vi "Set Batch Text.vi"(0 "VISA resource name":refnum<visa-resource-name>, 5 "Field Number (1)":i32=1 min=1 max=24, 7 "Field Title (\"\")":string, 9 "Field String (\"\")":string, 11 "error in (no error)":errorcluster) -> (4 "VISA resource name out":refnum<visa-resource-name>, 15 "error out":errorcluster)   [LabVIEW 2020, in "Yokogawa GX Series.lvlib"]
doc: "Sets the batch text.\n\nCommand: OBatText"
uses:
  <instrlib>/Yokogawa GX Series/Yokogawa GX Series.lvlib
panel:
  in  "Batch Group Number  (0: OFF)":i32(ring) items=["OFF", "1", "2", "3", "4", "5", "6", "7", "8", "9", "10", "11", "12"]
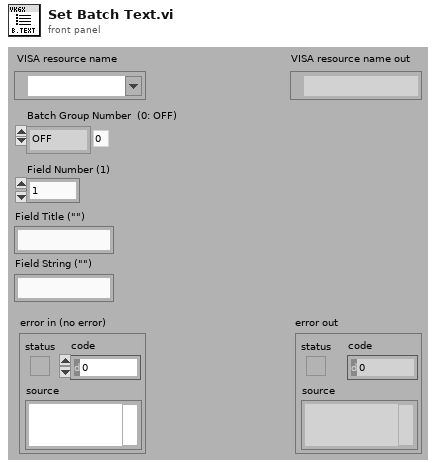
[diagram p1: front panel]
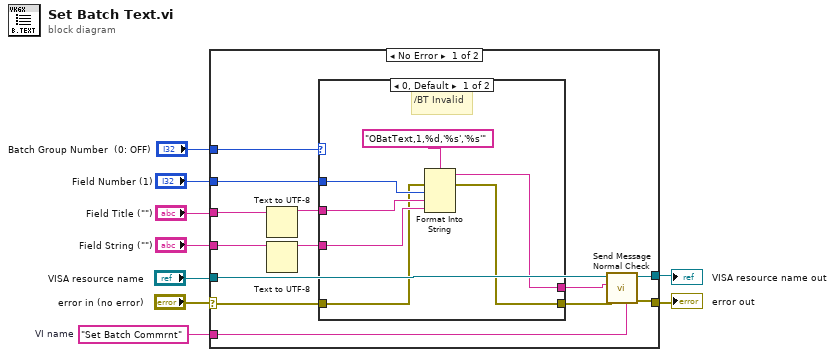
[diagram p0: block diagram]
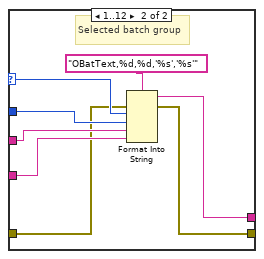
[diagram p2: hidden frame]
diagram:
  w8 = "Set Batch Commrnt"  # VI name
  n1 = case shown="No Error" "error in (no error)" {
    selector: "error in (no error)" -> [w12 w38]
    tunnel: "VISA resource name" -> [w22 w39]
    tunnel: w8 -> [w21 _]
    tunnel: [w20 w39] -> w7
    tunnel: [w19 w38] -> w6
    tunnel: "Field Number (1)" -> [w15 _]
    tunnel: "Field Title (\"\")" -> [w17 _]
    tunnel: "Field String (\"\")" -> [w18 _]
    tunnel: "Batch Group Number  (0: OFF)" -> [w16 _]
    frame No Error {
      n2 = Text to UTF-8(11:w17) -> (3:w14:string)  [unwired: 2 in, 1 out]
      n3 = Text to UTF-8(11:w18) -> (3:w13:string)  [unwired: 2 in, 1 out]
      n4 = case shown="0, Default" w16 {
        selector: w16 -> [_ w35]
        tunnel: [w29 w37] -> w11
        tunnel: [w28 w36] -> w10
        tunnel: w15 -> [w26 w33]
        tunnel: w14 -> [w25 w32]
        tunnel: w13 -> [w24 w31]
        tunnel: w12 -> [w23 w30]
        frame 0, Default {
          # "/BT Invalid"
          n5 = Format Into String(format string="OBatText,1,%d,'%s','%s'", error in=w23, w26, w25, w24) -> (resulting string=w28:string, error out=w29:errorcluster)  [unwired: 1 in]
        }
        frame 1..12 {
          # "Selected batch group"
          n6 = Format Into String(format string="OBatText,%d,%d,'%s','%s'", error in=w30, w35, w33, w32, w31) -> (resulting string=w36:string, error out=w37:errorcluster)  [unwired: 1 in]
        }
      }
      n7 = call <instrlib>:"Send Message Normal Check.vi"("Source (\"\")"=w21, "error in (no error)"=w11, "Send Message (\"\")"=w10, "VISA resource name"=w22) -> ("error out"=w19:errorcluster, "VISA resource name out"=w20:refnum<visa-resource-name>)  [unwired: 2 in, 4 out]
    }
    frame Error {
    }
  }
  "error out" <- w6
  "VISA resource name out" <- w7
